vi "Configure.vi"(8 "error in (no error)":errorcluster, 10 "Serial Settings":T1={"baud rate"=115200, "data bits"=8, "parity"=enum."None", "stop bits"=10, "flow control"=0} {"flow control" items=["None"=0, "XON/XOFF"=1, "RTS/CTS"=2, "DTR/DSR"=4]; "stop bits" items=["1.0"=10, "1.5"=15, "2.0"=20]; "data bits" min=5 max=8 step=1; "baud rate" items=["75"=75, "110"=110, "134"=134, "150"=150, "300"=300, "600"=600, "1200"=1200, "1800"=1800, "2400"=2400, "4800"=4800, "7200"=7200, "9600"=9600, "14400"=14400, "19200"=19200, "28800"=28800, "38400"=38400, "56000"=56000, "57600"=57600, "115200"=115200, "128000"=128000, "230400"=230400]}, 11 "ArduinoAIReal in":refnum<class "Arduino.lvclass">) -> (0 "error out":errorcluster, 3 "ArduinoAIReal out":refnum<class "Arduino.lvclass">)   [LabVIEW 2020, in "Arduino.lvlib" / "Arduino.lvclass"]
doc: "- configures VISA serial connection"
uses:
  Arduino.lvclass
  Arduino.lvclass/Arduino.ctl
  <vilib>/Instr/_visa.llb/VISA Configure Serial Port (Instr).vi
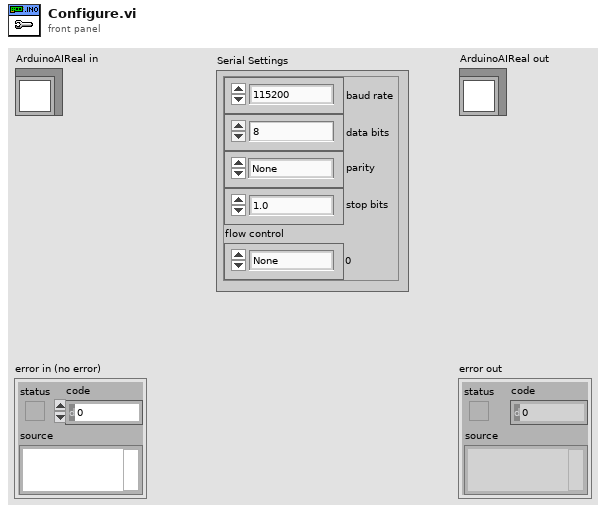
[diagram p1: front panel]
types:
  T1 = cluster{"baud rate":u32, "data bits":u16, "parity":enum16{"None", "Odd", "Even", "Mark", "Space"}, "stop bits":u16, "flow control":u16}
  T2 = cluster{"XON":enum16{"NUL", "SOH", "STX", "ETX", "EOT", "ENQ", "ACK", "BEL", "BS", "HT", "LF", "VT", "FF", "CR", "SO", "SI", "DLE", "DC1", "DC2", "DC3", "DC4", "NAK", "SYN", "ETB", "CAN", "EM", "SUB", "ESC", "FS", "GS", "RS", "US", "SP", "!", "\"", "#", "$", "%", "&", "'", "(", ")", "*", "+", ",", "- (-)", ".", "/", "0", "1", "2", "3", "4", "5", "6", "7", "8", "9", ":", ";", "<", "=", ">", "?", "@", "A", "B", "C", "D", "E", "F", "G", "H", "I", "J", "K", "L", "M", "N", "O", "P", "Q", "R", "S", "T", "U", "V", "W", "X", "Y", "Z", "[", "\\", "]", "^", "_", "`", "a", "b", "c", "d", "e", "f", "g", "h", "i", "j", "k", "l", "m", "n", "o", "p", "q", "r", "s", "t", "u", "v", "w", "x", "y", "z", "{", "|", "}", "~"}, "XOFF":enum16{"NUL", "SOH", "STX", "ETX", "EOT", "ENQ", "ACK", "BEL", "BS", "HT", "LF", "VT", "FF", "CR", "SO", "SI", "DLE", "DC1", "DC2", "DC3", "DC4", "NAK", "SYN", "ETB", "CAN", "EM", "SUB", "ESC", "FS", "GS", "RS", "US", "SP", "!", "\"", "#", "$", "%", "&", "'", "(", ")", "*", "+", ",", "- (-)", ".", "/", "0", "1", "2", "3", "4", "5", "6", "7", "8", "9", ":", ";", "<", "=", ">", "?", "@", "A", "B", "C", "D", "E", "F", "G", "H", "I", "J", "K", "L", "M", "N", "O", "P", "Q", "R", "S", "T", "U", "V", "W", "X", "Y", "Z", "[", "\\", "]", "^", "_", "`", "a", "b", "c", "d", "e", "f", "g", "h", "i", "j", "k", "l", "m", "n", "o", "p", "q", "r", "s", "t", "u", "v", "w", "x", "y", "z", "{", "|", "}", "~"}}
  T3 = enum16{"NUL", "SOH", "STX", "ETX", "EOT", "ENQ", "ACK", "BEL", "BS", "HT", "LF", "VT", "FF", "CR", "SO", "SI", "DLE", "DC1", "DC2", "DC3", "DC4", "NAK", "SYN", "ETB", "CAN", "EM", "SUB", "ESC", "FS", "GS", "RS", "US", "SP", "!", "\"", "#", "$", "%", "&", "'", "(", ")", "*", "+", ",", "- (-)", ".", "/", "0", "1", "2", "3", "4", "5", "6", "7", "8", "9", ":", ";", "<", "=", ">", "?", "@", "A", "B", "C", "D", "E", "F", "G", "H", "I", "J", "K", "L", "M", "N", "O", "P", "Q", "R", "S", "T", "U", "V", "W", "X", "Y", "Z", "[", "\\", "]", "^", "_", "`", "a", "b", "c", "d", "e", "f", "g", "h", "i", "j", "k", "l", "m", "n", "o", "p", "q", "r", "s", "t", "u", "v", "w", "x", "y", "z", "{", "|", "}", "~"}
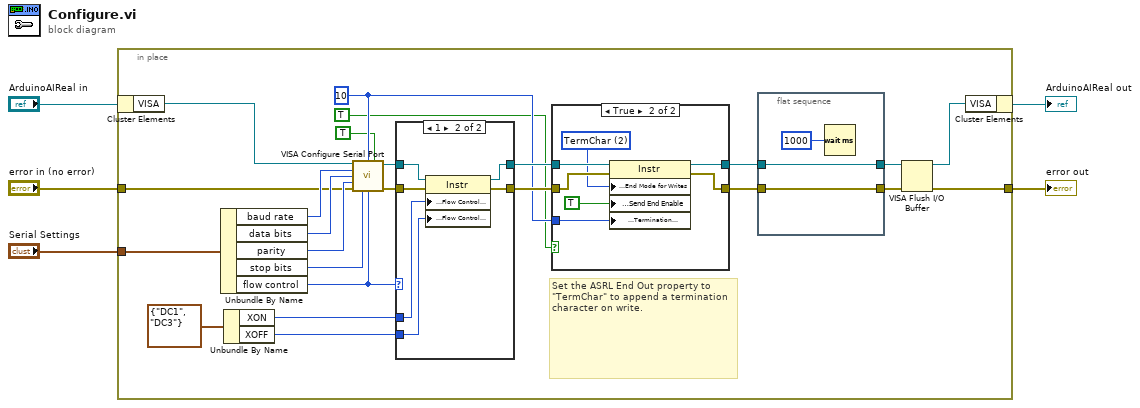
[diagram p0: block diagram]
diagram:
  n1 = in-place {
    in-place-border: "error in (no error)" -> [w10]
    in-place-border: [w9] -> w2
    in-place-border: "Serial Settings" -> [w6]
    w13 = u8 10 ("Termination Character")
    # "Set the ASRL End Out property to \"TermChar\" to append a termination character on write."
    n2 = in-place-cluster #1("ArduinoAIReal in") -> ("VISA"=w8:refnum<visa-resource-name>)
    n3 = Unbundle By Name(w6) -> ("baud rate"=w20:u32, "data bits"=w19:u16, "parity"=w18:enum16{"None", "Odd", "Even", "Mark", "Space"}, "stop bits"=w17:u16, "flow control"=w21:u16)
    n4 = Unbundle By Name(T2 {"XON"=enum."DC1", "XOFF"=enum."DC3"} ("XON/XOFF Characters")) -> ("XON"=w22:T3, "XOFF"=w23:T3)
    n5 = call-poly "VISA Configure Serial Port"("VISA resource name"=w8, "termination char\n(0xA = '\\n' = LF)"=w13, "Enable Termination\nChar (T)"=TRUE ("End Read on Termination Character?"), "baud rate (9600)"=w20, "data bits (8)"=w19, "parity (0:none)"=w18, "error in (no error)"=w10, "stop bits (10: 1 bit)"=w17, "flow control (0:none)"=w21) -> ("VISA resource name out"=w16:refnum<visa-resource-name>, "error out"=w15:errorcluster)  [unwired: 1 in, 4 out]
    n6 = case shown="1" w21 {
      tunnel: [w42 w49] -> w24
      tunnel: [w43 w48] -> w25
      tunnel: w15 -> [w42 w47]
      tunnel: w16 -> [w43 w46]
      tunnel: w22 -> [_ w45]
      tunnel: w23 -> [_ w44]
      frame Default {
      }
      frame 1 {
        n7 = property class="Instr"(reference=w46, error in=w47, "Serial Settings:Flow Control XON Character"=w45, "Serial Settings:Flow Control XOFF Character"=w44) -> (reference out=w48:refnum<visa-resource-name>, error out=w49:errorcluster)
      }
    }
    n8 = case shown="True" TRUE ("End Write on Termination Character?") {
      tunnel: w25 -> [w33 w41]
      tunnel: w24 -> [w34 w40]
      tunnel: [w33 w39] -> w26
      tunnel: [w34 w38] -> w27
      tunnel: w13 -> [_ w36]
      frame False {
      }
      frame True {
        w37 = u16 2 items=["None", "LastBit", "TermChar", "Break"] ("Serial Settings:Serial End Mode for Writes")
        n9 = property class="Instr"(reference=w41, error in=w40, "Serial Settings:End Mode for Writes"=w37, "Message Based Settings:Send End Enable"=TRUE, "Message Based Settings:Termination Character"=w36) -> (reference out=w39:refnum<visa-resource-name>, error out=w38:errorcluster)
      }
    }
    n10 = flat-sequence {
      tunnel: [w32] -> w28
      tunnel: w26 -> [w32]
      tunnel: [w31] -> w29
      tunnel: w27 -> [w31]
      frame #0 {
        n11 = Wait (ms)(milliseconds to wait=u32 1000) -> ()  [unwired: 1 out]
      }
    }
    n12 = VISA Flush I/O Buffer(VISA resource name=w28, error in (no error)=w29) -> (VISA resource name out=w7:refnum<visa-resource-name>, error out=w9:errorcluster)  [unwired: 1 in]
    n13 = in-place-cluster #1("VISA"=w7) -> (→"ArduinoAIReal out":refnum<class "Arduino.lvclass">)
  }
  "error out" <- w2
